vi "GUI_General_Camera.vi"() -> ()   [LabVIEW 2013]
uses:
  <vilib>/vision/NI_Vision_Development_Module.lvlib
  Shared/MySQL/Preset Query Enum.ctl
  <vilib>/Utility/miscctls.llb/LVRectTypeDef.ctl
panel:
  in  "resize":bool
  in  "Tab Control":T1(tab)
  in  "Maximize!!":bool
  out "Max Counts":dbl(slide) scale=0.0..256.0
  in  "triggerdelay":dbl
  in  "trigger":bool
  in  "save":bool
  in  "exposure":dbl=0.52 caption="Exposure"
  in  "gain":dbl
  in  "shotnumber":i32=354
  in  "autoscale":bool
  in  "LogArray":bool
  in  "beep if sat.":bool
  in  "sat level":sgl=255.0
  in  "lowpass":bool
  in  "Size & Tolerance":T2={"X Size"=5, "Y Size"=5, "% Tolerance"=10}
  in  "hide controls":bool
  in  "ROI.OffsetY":dbl
  in  "ROI.OffsetX":dbl
  in  "ROI.Height":dbl
  in  "ROI.Width":dbl
  in  "MaxGUIPixel":dbl
  out "Centroid":cluster{"X Centroid":sgl, "Y Centroid":sgl} {"Y Centroid" format="%.2f"; "X Centroid" format="%.2f"}
  out "Y Resolution":i32
  out "X Resolution":i32
  out "Mean Value":sgl format="%.2f"
  out "GUIBinning":dbl
  in  "Target.Y":dbl
  in  "Target.X":dbl
  in  "draw Xhair":bool
  in  "size 2":cluster{"xhair size":dbl, "xhair size 2":dbl}={"xhair size"=20.0, "xhair size 2"=20.0} {"xhair size 2" min=0.0 max=0.0; "xhair size" min=0.0 max=0.0}
  out "Mean Value 2":sgl(graph)
  out "histogram":T3(graph)
  out "lineout":cluster{"x0":sgl, "dx":sgl, "Pixels Line":sgl[]}(graph)
  out "MaxCounts":dbl
  in  "FWHMx":dbl
  in  "FWHMy":dbl
  out "MeanCounts":dbl
  out "FWHMx (um)":dbl
  out "FWHMy (um)":dbl
  in  "SpatialCalibration":dbl
  in  "Analysis":bool
  out "analysis error":errorcluster
  out "top":i16
  out "left":i16
  out "Zoom changed":bool
  out "Zoom old":cluster{"X":sgl, "Y":sgl}
  out "ratio(h)":bool=TRUE
  out "fixsize":bool
  out "Change Ratio":cluster{"X":sgl, "Y":sgl}={"X"=1.6671598, "Y"=0.6151203}
  out "old Panel Bounds":T4={"Left"=105, "Top"=80, "Right"=781, "Bottom"=662}
  out "error (h)":bool
  in  "Main Tap":enum32{"IMAQ", "Network", "Internal", "Array"}(tab)
  out "Image (IMAQ)":T5(plugin-control)
  out "local Port":u16=65401
  out "Remote Host":string="192.168.10.157"
  out "port or service name":u16=65400
  in  "timeout ms (slow resp)":i32=500
  in  "reset":bool
  out "All Devices (h)":string[](array[string])
  out "centroidy":dbl
  out "fast ID (h)":refnum<k16>
  out "slow ID (h)":refnum<k16>
  out "error out":errorcluster
  out "connections (hidden)":variant[](array[variant])=[variant(refnum<k16> refnum), variant(refnum<k16> refnum)]
  in  "time to wait (main loop)":i32=200
  in  "time to wait (TCP)":i32=10
  out "Data String":string="exposure,0.520000\r\ntrigger,off\r\nsave,off\r\ngain,0.000000\r\n"
  in  "send":bool
  in  "localsavingpath":path
  out "centroidy":dbl
  out "Image (array)":dbl[][](graph)
  out "Device Name (h)":string="FakeCam1"
  out "stop":bool
  out "error message":string
  out "image connection":bool
  out "data connection ok":bool
  # "Trigger"
  # "Save"
  # "Data"
  # "Image"
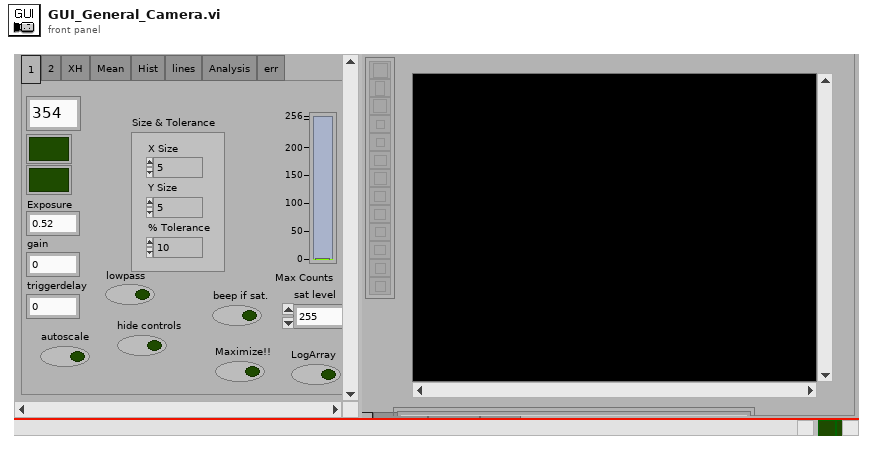
[diagram p1: front panel]
types:
  T1 = enum32{"1", "2", "XH", "Mean", "Hist", "lines", "Analysis", "err"}
  T2 = cluster{"X Size":i32, "Y Size":i32, "% Tolerance":i32}
  T3 = cluster{"Starting Value":sgl, "Incremental Value":sgl, "Histogram":u32[]}
  T4 = typedef "LVRectTypeDef.ctl" = cluster{"Left":i16, "Top":i16, "Right":i16, "Bottom":i16}
  T5 = typedef "IMAQ Image.ctl" = refnum<image>
  T6 = enum16{"Grayscale", "Binary", "Gradient", "Rainbow", "Temperature", "User Defined"}
  T7 = typedef "Preset Query Enum.ctl" = enum16{"Get Locations", "Get all IPs and MACs", "Get classes", "Get expt variables to set at scanstart for particular device", "Get expt devices and variables with start values", "Get expt devices and variables (with data to get)", "Get expt devices with data to get", "Get Expt devices and GUIs", "Get all devices basic properties", "Get Virtual Devices Core Info", "Get Expt names", "Get experiment basic properties", "Get experiment alarm variables", "Get MC Ports", "Get device network comm port", "Get devicetype lvclass path", "Get basic device properties", "Get Init Order", "Get all setable variables of a device", "Get device variable aliases", "Get force values of all settable variables", "Get all variables of a devicetype", "Get all variables of a device", "Get plotter details", "Get Saved Scans", "Get Scan Info", "GetGeneralGUIs", "Get expt for plotter", "Get plotter IDs from expt", "Get all devices", "Get all Virtual Devices", "Get all aliases", "Get variable and device info for Virtual Device", "GetItemLocatorIP", "Get IPs for GUIs", "Get DeviceType from Device", "GetLocalPortRange", "GetDevicePresetVariables", "Get Device Configuration", "GetAllPresetNames", "GetAllConfigurationNames", "GetPresetDeviceNames"}
  T8 = cluster{"Left":i32, "Top":i32, "Right":i32, "Bottom":i32}
  T9 = enum32{"Invalid", "Standard", "Closed", "Hidden", "Minimized", "Maximized"}
  T10 = typedef "Image Type" = u32
  T11 = cluster{"Global Rectangle":i32[], "Contours":cluster{"Contour Type":u32, "ROI Type":u32, "Points":i32[]}[]}
  T12 = typedef "EventTypDef.ctl" = refnum<user-event>
  T13 = typedef "LVBoundsTypeDef.ctl" = cluster{"Width":u32, "Height":u32}
  T14 = typedef "ROI Descriptor" = cluster{"Global Rectangle":i32[], "Contours":cluster{"ID":enum32{"External", "Internal"}, "Type":u32, "Coordinates":i32[]}[]}
  T15 = typedef "IMAQ Line" = cluster{"Start X":i32, "Start Y":i32, "End X":i32, "End Y":i32}
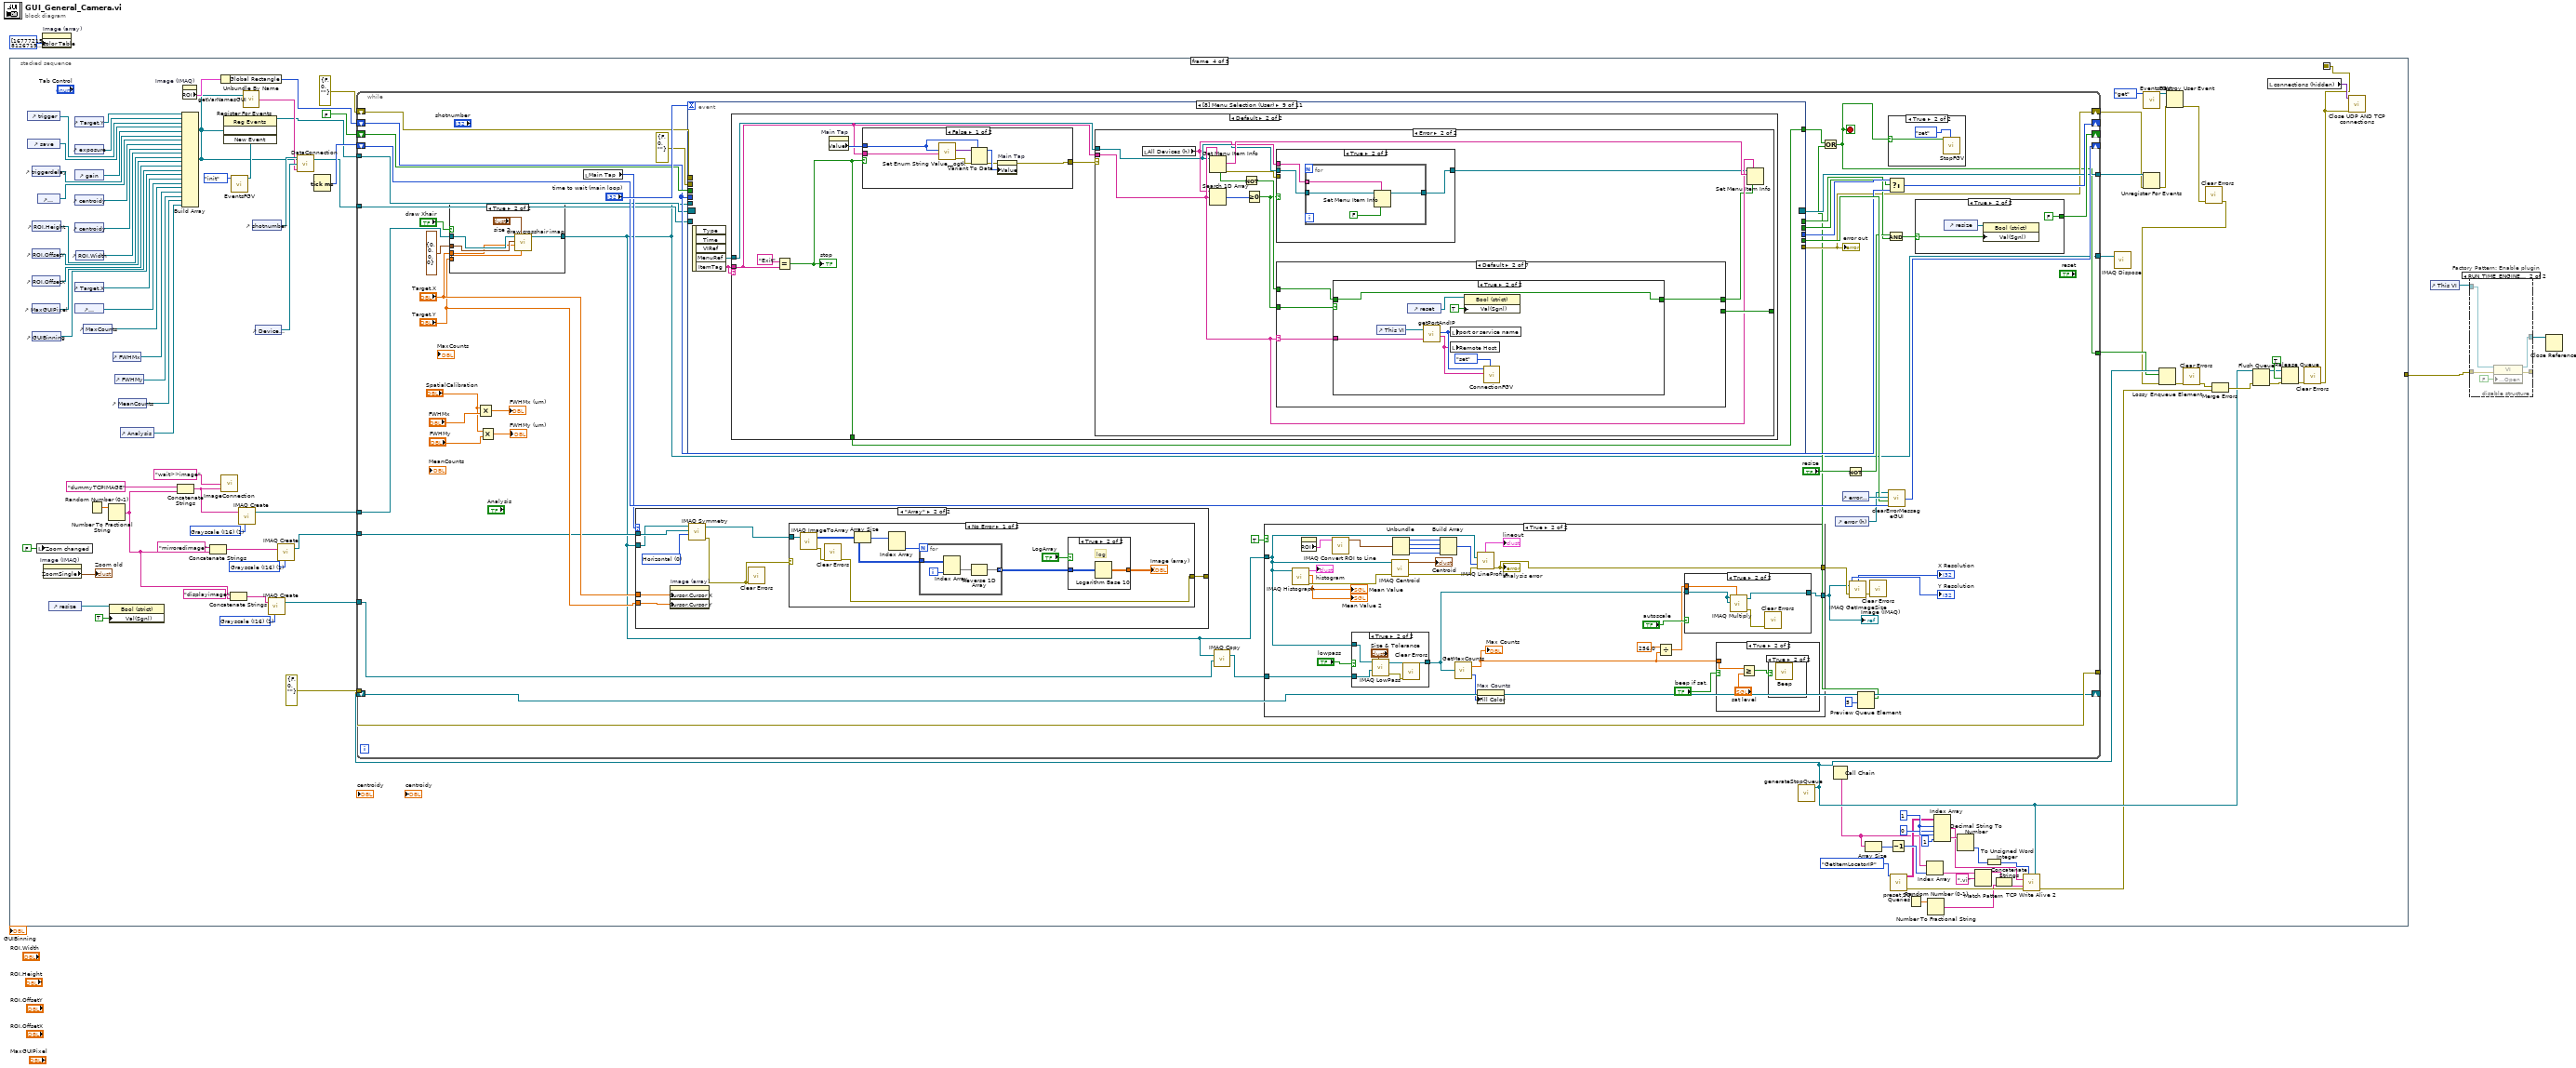
[diagram p0: block diagram]
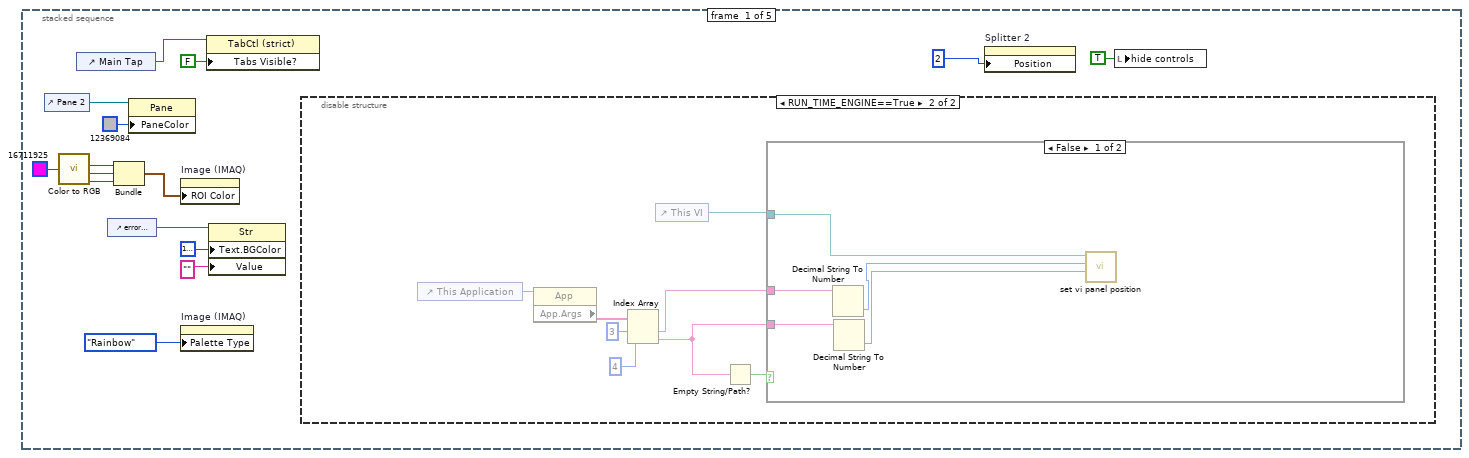
[diagram p3: hidden frame]
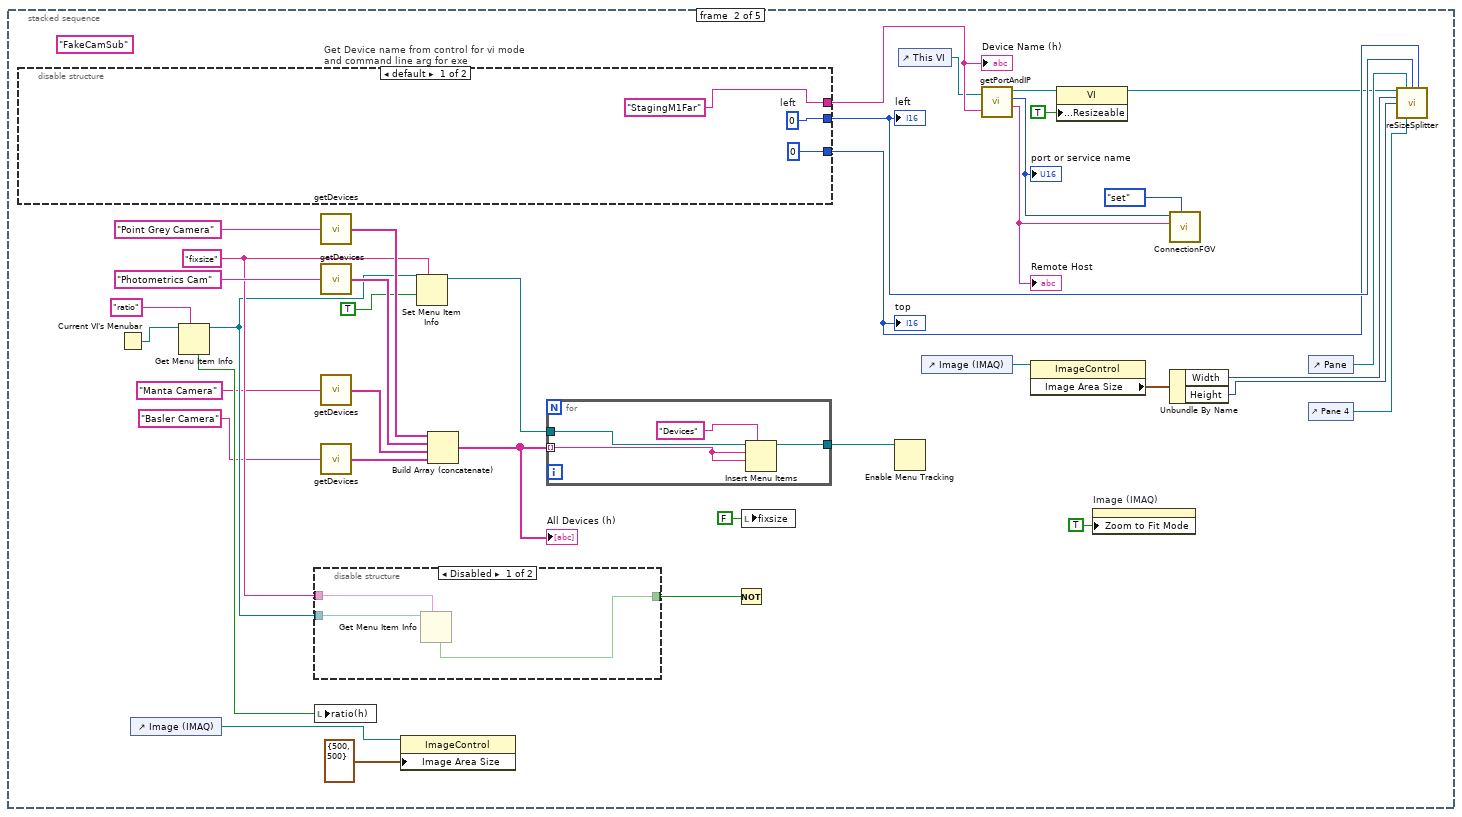
[diagram p6: hidden frame]
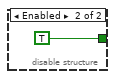
[diagram p7: hidden frame]
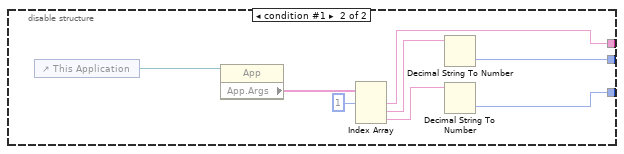
[diagram p8: hidden frame]
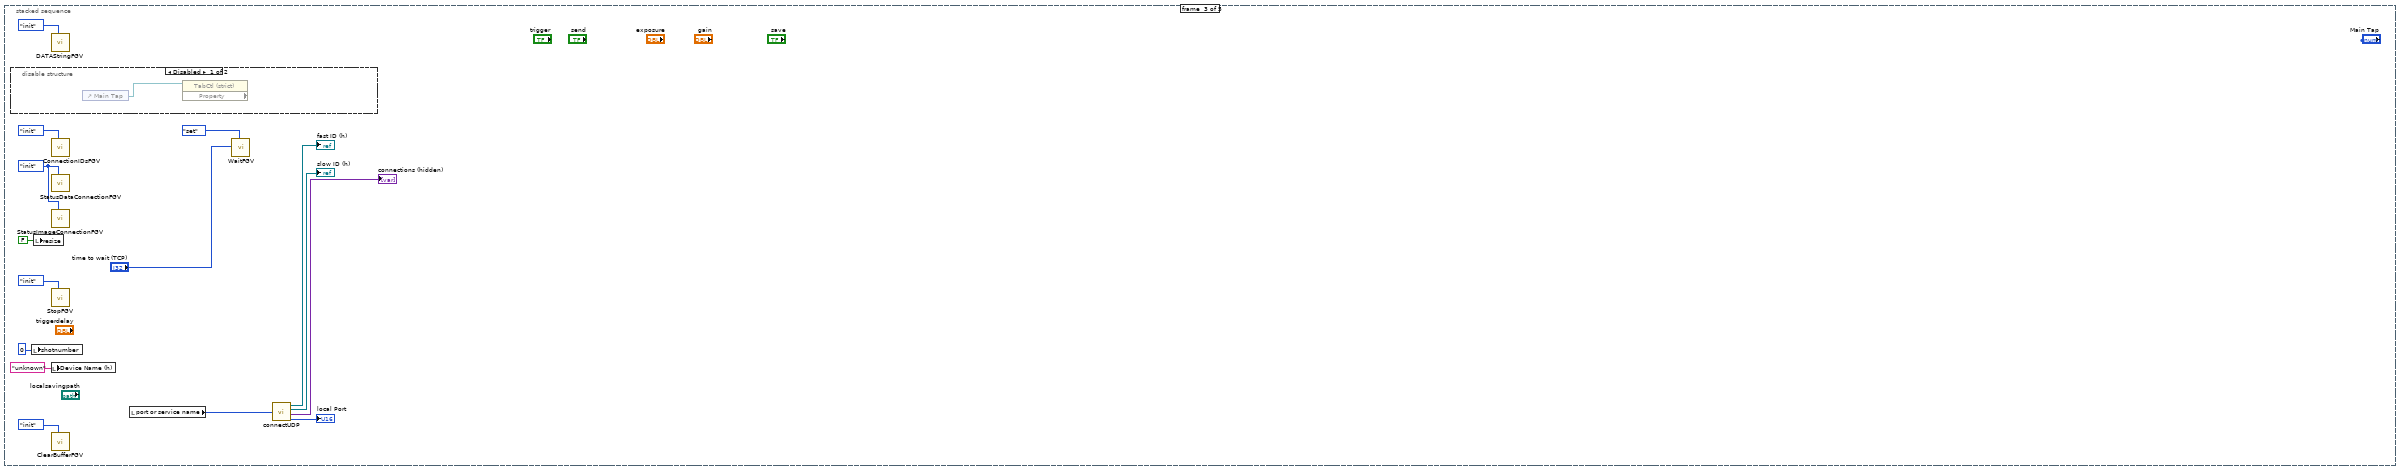
[diagram p9: hidden frame]
diagram:
  n1 = stacked-sequence {
    seq-local: [_ _ _ w140 _] -> [_ _ _ _ w550]
    tunnel: [_ _ _ _ w550] -> w2
    frame #0 {
      n2 = control-ref of="Pane 2"() -> (w14:refnum<vi>)
      n3 = call <vilib>:"Color to RGB.vi"("Color"=u32 16711925) -> ("R"=w10:u8, "G"=w9:u8, "B"=w8:u8)  [unwired: 1 out]
      n4 = control-ref of="Main Tap"() -> (w19:refnum<vi>)
      n5 = control-ref of="error message"() -> (w16:refnum<vi>)
      n6 = Bundle("R"=w10, "G"=w9, "B"=w8) -> (w7:cluster{"R":u8, "G":u8, "B":u8})  [unwired: 1 in]
      n7 = property class="Pane"(reference=w14, "PaneColor"=u32 12369084) -> ()  [unwired: 1 in, 2 out]
      n8 = property on="Image (IMAQ)" class="ImageControl"("ROI Color"=w7) -> ()  [unwired: 2 in, 2 out]
      n9 = property on="Image (IMAQ)" class="ImageControl"("Palette Type"=T6."Rainbow" ("Palette:Palette Type")) -> ()  [unwired: 2 in, 2 out]
      n10 = property class="TabCtl (strict)"(reference=w19, "Tabs Visible?"=FALSE) -> ()  [unwired: 1 in, 2 out]
      n11 = property class="Str"(reference=w16, "Text.BGColor"=u32 16777238, "Value"="") -> ()  [unwired: 1 in, 2 out]
      n12 = disable-structure shown="RUN_TIME_ENGINE==True" {
        frame condition #0 (active) {
        }
        frame condition #1 {
          n13 = control-ref of="This Application"() -> (w20:refnum<vi>)
          n14 = property class="App"(reference=w20) -> ("App.Args"=w27:string[])  [unwired: 1 in, 2 out]
          n15 = Index Array(array=w27, index #1=3 ("index"), index #2=4 ("index")) -> (element #1=w24:string, element #2=w23:string)
          n16 = control-ref of="This VI"() -> (w21:refnum<vi>)
          n17 = Empty String/Path?(string/path=w23) -> (empty?=w22:bool)
          n18 = case shown="False" w22 {
            tunnel: w24 -> [w32 _]
            tunnel: w21 -> [w28 _]
            tunnel: w23 -> [w29 _]
            frame False {
              n19 = Decimal String To Number(string=w32) -> (number=w31:i32)  [unwired: 2 in, 1 out]
              n20 = Decimal String To Number(string=w29) -> (number=w30:i32)  [unwired: 2 in, 1 out]
              n21 = call "set vi panel position.vi"("top"=w30, "left"=w31, "This VI"=w28) -> ()  [unwired: 7 in, 2 out]
            }
            frame True {
            }
          }
        }
      }
      n22 = property on="Splitter 2" class="Splitter"("Position"=2 ("Position:Left")) -> ()  [unwired: 2 in, 2 out]
      n23 = local write "hide controls"(TRUE ("hide controls")) -> ()
    }
    frame #1 {
      (unwired) "FakeCamSub" ("Device Class")
      w42 = "fixsize" ("item tag")
      n24 = disable-structure "Get Device name from control for vi mode\nand command line arg for exe" shown="default" {
        disable-tunnel: ["StagingM1Far" ("Device Name for vi mode") w86] -> w57
        disable-tunnel: [w80 w83] -> w62
        disable-tunnel: [i16 0 ("left") w82] -> w61
        frame condition #0 (active) {
          w80 = i16 0  # left
        }
        frame condition #1 {
          n25 = control-ref of="This Application"() -> (w89:refnum<vi>)
          n26 = property class="App"(reference=w89) -> ("App.Args"=w88:string[])  [unwired: 1 in, 2 out]
          n27 = Index Array(array=w88, index #1=1 ("index")) -> (element #1=w86:string, element #2=w85:string, element #3=w84:string)  [unwired: 2 in]
          n28 = Decimal String To Number(string=w85) -> (number=w83:i32)  [unwired: 2 in, 1 out]
          n29 = Decimal String To Number(string=w84) -> (number=w82:i32)  [unwired: 2 in, 1 out]
        }
      }
      "Device Name (h)" <- w57
      "left" <- w62
      "top" <- w61
      n30 = Current VI's Menubar() -> (w64:refnum<k9>)
      n31 = control-ref of="Image (IMAQ)"() -> (w45:refnum<vi>)
      n32 = Get Menu Item Info(7:"ratio" ("item tag"), 11:w64) -> (3:w41:refnum<k9>, 4:w63:bool)  [unwired: 1 in, 5 out]
      n33 = disable-structure shown="Disabled" {
        disable-tunnel: [w73 TRUE] -> w60
        disable-tunnel: w42 -> [w72 _]
        disable-tunnel: w41 -> [w71 _]
        frame Disabled {
          n34 = Get Menu Item Info(7:w72, 11:w71) -> (4:w73:bool)  [unwired: 1 in, 6 out]
        }
        frame Enabled {
        }
      }
      n35 = local write "ratio(h)"(w63) -> ()
      n36 = call "getDevices.vi"("Device Class"="Point Grey Camera") -> ("All Devices"=w48:string[])
      n37 = call "getDevices.vi"("Device Class"="Photometrics Cam") -> ("All Devices"=w47:string[])
      n38 = call "getDevices.vi"("Device Class"="Manta Camera") -> ("All Devices"=w37:string[])
      n39 = call "getDevices.vi"("Device Class"="Basler Camera") -> ("All Devices"=w35:string[])
      n40 = property class="ImageControl"(reference=w45, "Image Area Size"=cluster{"Width":u32, "Height":u32} {"Width"=500, "Height"=500} ("Image Area:Size:All Elements")) -> ()  [unwired: 1 in, 2 out]
      n41 = Set Menu Item Info(7:w42, 9:TRUE ("enabled"), 11:w41) -> (3:w40:refnum<k9>)  [unwired: 4 in, 1 out]
      n42 = Build Array (concatenate)(w48, w47, w37, w35) -> (w46:string[])
      "All Devices (h)" <- w46
      n43 = for {
        tunnel: w40 -> [w78]
        tunnel: [w77] -> w58
        tunnel: w46 -> [w75] mode=indexing
        n44 = Insert Menu Items(5:"Devices" ("menu tag"), 7:w75, 8:w75, 9:w78) -> (3:w77:refnum<k9>)  [unwired: 2 in, 2 out]
      }
      n45 = Not(x=w60) -> ()  [unwired: 1 out]
      n46 = local write "fixsize"(FALSE ("fixsize")) -> ()
      n47 = Enable Menu Tracking(4:w58) -> ()  [unwired: 2 in, 2 out]
      n48 = control-ref of="This VI"() -> (w56:refnum<vi>)
      n49 = control-ref of="Image (IMAQ)"() -> (w70:refnum<vi>)
      n50 = call "getPortAndIP.vi"("This Vi"=w56, "Device Name"=w57) -> ("reference out"=w55:refnum<vi>, "port or service name"=w52:u16, "Remote Host"=w51:string)  [unwired: 1 in]
      "port or service name" <- w52
      "Remote Host" <- w51
      n51 = property class="ImageControl"(reference=w70) -> ("Image Area Size"=w69:cluster{"Width":u32, "Height":u32})  [unwired: 1 in, 2 out]
      n52 = property class="VI"(reference=w55, "Front Panel.Resizeable"=TRUE ("Front Panel Window:Resizable")) -> (reference out=w54:refnum<vi>)  [unwired: 1 in, 1 out]
      n53 = property on="Image (IMAQ)" class="ImageControl"("Zoom to Fit Mode"=TRUE) -> ()  [unwired: 2 in, 2 out]
      n54 = call "ConnectionFGV.vi"("command"=enum16{"get", "set", "init"}."set", "Remote Host in"=w51, "port or service name in"=w52) -> ()  [unwired: 7 in, 2 out]
      n55 = Unbundle By Name(w69) -> ("Width"=w68:u32, "Height"=w67:u32)
      n56 = control-ref of="Pane"() -> (w66:refnum<vi>)
      n57 = control-ref of="Pane 4"() -> (w59:refnum<vi>)
      n58 = call "reSizeSplitter.vi"("this vi"=w54, "pane"=w66, "left"=w62, "top"=w61, "Width"=w68, "Height"=w67, "pane2"=w59) -> ()  [unwired: 8 in, 1 out]
    }
    frame #2 {
      w100 = enum16{"get", "set", "init"}."init" ("Command")
      n59 = disable-structure shown="Disabled" {
        frame Disabled {
          n60 = control-ref of="Main Tap"() -> (w105:refnum<vi>)
          n61 = property class="TabCtl (strict)" props=[](reference=w105) -> ()  [unwired: 1 in, 3 out]
        }
        frame Enabled {
        }
      }
      n62 = local write "shotnumber"(0 ("shotnumber")) -> ()
      n63 = local write "resize"(FALSE ("resize")) -> ()
      n64 = call "DATAStringFGV.vi"("Command"=enum16{"get", "set", "init"}."init") -> ()  [unwired: 9 in, 2 out]
      n65 = call "ConnectionIDsFGV.vi"("Command"=enum16{"add", "get", "init"}."init") -> ()  [unwired: 10 in, 1 out]
      n66 = call "StatusDataConnectionFGV.vi"("Command"=w100) -> ()  [unwired: 10 in, 1 out]
      n67 = call "StatusImageConnectionFGV.vi"("Command"=w100) -> ()  [unwired: 10 in, 1 out]
      n68 = call "StopFGV.vi"("Command"=enum16{"set", "get", "init"}."init") -> ()  [unwired: 9 in, 2 out]
      n69 = local write "Device Name (h)"("unknown" ("Device Name")) -> ()
      n70 = call "ClearBufferFGV.vi"("Command"=enum16{"set", "get", "init"}."init") -> ()  [unwired: 10 in, 1 out]
      n71 = local read "port or service name"() -> (w102:u16)
      n72 = call "WaitFGV.vi"("Command"=enum16{"get", "set", "init"}."set", "milliseconds to wait"="time to wait (TCP)") -> ()  [unwired: 9 in, 1 out]
      n73 = call "connectUDP.vi"("port or service name NOT USED"=w102) -> ("fast ID (h)"=→"fast ID (h)":refnum<k16>, "slow ID (h)"=→"slow ID (h)":refnum<k16>, "connections (hidden)"=→"connections (hidden)":variant[], "local Port"=→"local Port":u16)
    }
    frame #3 {
      w110 = T10 1 items=["Grayscale (U8)", "Grayscale (I16)", "Grayscale (SGL)", "Complex (CSG)", "RGB (U32)", "HSL (U32)", "RGB (U64)", "Grayscale (U16)"] ("Image Type")
      w114 = T10 1 items=["Grayscale (U8)", "Grayscale (I16)", "Grayscale (SGL)", "Complex (CSG)", "RGB (U32)", "HSL (U32)", "RGB (U64)", "Grayscale (U16)"] ("Image Type")
      w129 = 1 ("index (row)")
      w196 = T10 1 items=["Grayscale (U8)", "Grayscale (I16)", "Grayscale (SGL)", "Complex (CSG)", "RGB (U32)", "HSL (U32)", "RGB (U64)", "Grayscale (U16)"] ("Image Type")
      n74 = control-ref of="trigger"() -> (w189:refnum<vi>)
      n75 = control-ref of="save"() -> (w187:refnum<vi>)
      n76 = control-ref of="triggerdelay"() -> (w185:refnum<vi>)
      n77 = control-ref of="ROI.OffsetY"() -> (w159:refnum<vi>)
      n78 = control-ref of="ROI.OffsetX"() -> (w158:refnum<vi>)
      n79 = control-ref of="MaxGUIPixel"() -> (w157:refnum<vi>)
      n80 = control-ref of="ROI.Height"() -> (w160:refnum<vi>)
      n81 = control-ref of="GUIBinning"() -> (w156:refnum<vi>)
      n82 = local write "Zoom changed"(FALSE ("Zoom changed")) -> ()
      n83 = control-ref of="localsavingpath"() -> (w181:refnum<vi>)
      n84 = property on="Image (IMAQ)" class="ImageControl"() -> ("ZoomSingle"=→"Zoom old":cluster{"X":sgl, "Y":sgl})  [unwired: 2 in, 2 out]
      n85 = control-ref of="resize"() -> (w171:refnum<vi>)
      n86 = control-ref of="Target.Y"() -> (w154:refnum<vi>)
      n87 = control-ref of="exposure"() -> (w188:refnum<vi>)
      n88 = control-ref of="gain"() -> (w186:refnum<vi>)
      n89 = control-ref of="centroidy"() -> (w180:refnum<vi>)
      n90 = control-ref of="centroidy"() -> (w174:refnum<vi>)
      n91 = control-ref of="Target.X"() -> (w155:refnum<vi>)
      n92 = control-ref of="SpatialCalibration"() -> (w153:refnum<vi>)
      n93 = control-ref of="ROI.Width"() -> (w161:refnum<vi>)
      n94 = control-ref of="MaxCounts"() -> (w152:refnum<vi>)
      n95 = Random Number (0-1)() -> (number: 0 to 1=w194:dbl)
      n96 = Number To Fractional String(number=w194) -> (F-format string=w106:string)  [unwired: 3 in]
      n97 = property class="Bool (strict)"(reference=w171, "Val(Sgnl)"=TRUE ("Value (Signaling)")) -> ()  [unwired: 1 in, 2 out]
      n98 = control-ref of="FWHMx"() -> (w151:refnum<vi>)
      n99 = control-ref of="FWHMy"() -> (w150:refnum<vi>)
      n100 = control-ref of="MeanCounts"() -> (w149:refnum<vi>)
      n101 = control-ref of="Analysis"() -> (w148:refnum<vi>)
      n102 = Concatenate Strings("dummyTCPIMAGE" ("Image Name"), w106) -> (w192:string)
      n103 = Build Array(w154, w188, w189, w187, w186, w185, w181, w180, w174, w161, w160, w159, w158, w157, w156, w155, w153, w152, w151, w150, w149, w148) -> (w168:refnum<vi>[])
      n104 = property on="Image (IMAQ)" class="ImageControl"() -> ("ROI"=w179:T11)  [unwired: 2 in, 2 out]
      n105 = Concatenate Strings("mirroredimage" ("string"), w106) -> (w112:string)
      n106 = Unbundle By Name(w179) -> ("Global Rectangle"=w178:i32[])
      n107 = call "ImageConnection.vi"("Image Name"=w192, "Image Subscriber list"="wait>>image") -> ()  [unwired: 2 in]
      n108 = Concatenate Strings("displayimage" ("string"), w106) -> (w108:string)
      n109 = call "EventsFGV.vi"("Command"=enum16{"get", "init"}."init") -> ("New Event"=w169:T12)  [unwired: 9 in, 1 out]
      n110 = register-events(w168, w169) -> (reference out=w167:refnum<event-registration>)  [unwired: 2 in, 1 out]
      n111 = call "IMAQ Create"("Image Name"=w192, "Image Type"=w196) -> ("New Image"=w195:T5)  [unwired: 3 in, 1 out]
      n112 = call "getVarNamesGUI.vi"("Array"=w168) -> ("String"=w173:string)  [unwired: 1 in]
      n113 = control-ref of="shotnumber"() -> (w176:refnum<vi>)
      n114 = control-ref of="Device Name (h)"() -> (w175:refnum<vi>)
      n115 = call "IMAQ Create"("Image Name"=w108, "Image Type"=w110) -> ("New Image"=w107:T5)  [unwired: 3 in, 1 out]
      n116 = call "IMAQ Create"("Image Name"=w112, "Image Type"=w114) -> ("New Image"=w111:T5)  [unwired: 3 in, 1 out]
      n117 = call "DataConnection.vi"("Subscriber list"=w173, "Device Name (h)"=w175, "shotnumber"=w176) -> ()
      n118 = Tick Count (ms)() -> (millisecond timer value=w182:u32)
      n119 = call "generateStopQueue.vi"() -> ("STOP Queue out"=w123:refnum<queue>)  [unwired: 10 in, 1 out]
      n120 = while {
        shift-right: [w226] -> w164
        shift-left: errorcluster {"status"=FALSE, "code"=0, "source"=""} ("error out") -> [w246]
        tunnel: w195 -> [w225]
        tunnel: [w201] -> w197
        tunnel: w168 -> [w233]
        shift-right: [w232] -> _
        shift-left: FALSE -> [w245]
        shift-right: [w244] -> _
        shift-left: w182 -> [w243]
        shift-right: [w238] -> _
        shift-left: w178 -> [w237]
        tunnel: w167 -> [w234]
        tunnel: [w227] -> w166
        tunnel: errorcluster {"status"=FALSE, "code"=0, "source"=""} ("error out") -> [w213]
        tunnel: [w213] -> _
        tunnel: [w209] -> w120
        shift-right: [w212] -> _
        shift-left: w123 -> [w214]
        tunnel: w111 -> [w207]
        tunnel: w107 -> [w200]
        stop <- w209 stop-if-true
        n121 = case shown="True" "draw Xhair" {
          tunnel: "Target.Y" -> [_ w291]
          tunnel: "Target.X" -> [_ w292]
          tunnel: w225 -> [w289 w295]
          tunnel: [w289 w293] -> w201
          tunnel: T8 {"Left"=0, "Top"=0, "Right"=0, "Bottom"=0} ("Bounding Rectangle") -> [_ w294]
          frame False {
          }
          frame True {
            n122 = call "draw crosshair imaq.vi"(6:w291, "clear overlay"="size 2", "Crosshair"=w292, "Bounding Rectangle"=w294, "image in"=w295) -> ("image out"=w293:T5)  [unwired: 5 in, 1 out]
          }
        }
        n123 = Multiply(x="SpatialCalibration", y="FWHMx") -> (x*y=→"FWHMx (um)":dbl)
        n124 = Multiply(x="SpatialCalibration", y="FWHMy") -> (x*y=→"FWHMy (um)":dbl)
        n125 = local read "Main Tap"() -> (w240:enum32{"IMAQ", "Network", "Internal", "Array"})
        n126 = case shown="\"Array\"" w240 {
          tunnel: w201 -> [_ w306]
          tunnel: "Target.X" -> [_ w309]
          tunnel: "Target.Y" -> [_ w308]
          tunnel: w207 -> [_ w307]
          tunnel: [_ w302] -> _
          frame "IMAQ", Default {
          }
          frame "Array" {
            w305 = u32 0 items=["Horizontal", "Vertical", "Central", "1st Diagonal", "2nd Diagonal"] ("Type of Symmetry")
            n127 = property on="Image (array)" class="IntGraph (strict)"("Cursor.Cursor X"=w309, "Cursor.Cursor Y"=w308) -> ()  [unwired: 2 in, 2 out]
            n128 = call "IMAQ Symmetry"("Type of Symmetry"=w305, "Image Dst"=w307, "Image Src"=w306) -> ("error out"=w303:errorcluster, "Image Dst Out"=w304:T5)  [unwired: 2 in]
            n129 = call <vilib>:"Clear Errors.vi"("error in (no error)"=w303) -> ()  [unwired: 6 in, 1 out]
            n130 = case shown="No Error" w303 {
              tunnel: w304 -> [w311 _]
              tunnel: [w310 _] -> w302
              frame No Error {
                n131 = call "IMAQ ImageToArray"("Image"=w311) -> ("error out"=w318:errorcluster, "Image Pixels (I16)"=w312:i16[][])  [unwired: 3 in, 3 out]
                n132 = call <vilib>:"Clear Errors.vi"("error in (no error)"=w318) -> ("error out"=w310:errorcluster)  [unwired: 6 in]
                n133 = Array Size(array=w312) -> (size(s)=w317:i32[])
                n134 = Index Array(array=w317) -> (element #2=w316:i32)  [unwired: 2 in, 1 out]
                n135 = for {
                  N: w316 -> [_]
                  tunnel: w312 -> [w325]
                  tunnel: [w323] -> w314 mode=indexing
                  i -> [w322]
                  n136 = Index Array(array=w325, index (col)=w322) -> (element=w324:i16[])  [unwired: 1 in]
                  n137 = Reverse 1D Array(array=w324) -> (reversed array=w323:i16[])
                }
                n138 = case shown="True" "LogArray" {
                  tunnel: w314 -> [w319 w321]
                  tunnel: [w319 w320] -> w313
                  frame False {
                  }
                  frame True {
                    # "log"
                    n139 = Logarithm Base 10(1:w321) -> (0:w320:dbl[][])
                  }
                }
                "Image (array)" <- w313
              }
              frame Error {
              }
            }
          }
        }
        n140 = event shown="[8] Menu Selection (User)" {
          selector: w234 -> [_ _ _ _ _ _ _ _ _ _ _]
          dyn-events: [_ _ _ _ _ _ _ _ _ _ _] -> w227
          timeout: "time to wait (main loop)" -> [_ _ _ _ _ _ _ _ _ _ _]
          tunnel: [w331 _ _ _ _ _ _ w449 _ _ _] -> w226
          tunnel: errorcluster {"status"=FALSE, "code"=0, "source"=""} ("error out") -> [w333 _ _ _ _ _ _ _ _ _ _]
          tunnel: w246 -> [_ _ _ _ _ _ _ w449 _ _ _]
          tunnel: [TRUE _ _ _ _ _ _ _ _ _ _] -> w241
          tunnel: [_ _ _ _ _ _ _ _ w452 _ _] -> w211
          tunnel: w245 -> [_ _ _ _ _ _ _ _ _ _ _]
          tunnel: [_ w341 w353 TRUE _ _ _ _ _ _ _] -> w229
          tunnel: [_ _ _ _ _ _ _ _ _ _ w526] -> w239
          tunnel: w237 -> [_ _ _ _ _ _ _ _ _ _ w527]
          tunnel: [_ _ _ _ _ _ _ _ _ _ w525] -> w236
          tunnel: w201 -> [_ _ _ _ _ _ w393 _ _ _ w528]
          tunnel: w233 -> [_ _ _ _ _ w383 _ _ _ _ _]
          event Value Change {
            n141 = event-data() -> ("CtlRef"=w328:refnum<vi>, "NewVal"=w327:variant)  [unwired: 1 in, 3 out]
            n142 = call "SendCommandEvent.vi"("timeout ms (slow resp)"="timeout ms (slow resp)", "error out 2"=w333, "NewVal"=w327, "CtlRef"=w328) -> ("error out"=w331:errorcluster, "error (h)"=→"error (h)":bool, "error message"=→"error message":string)  [unwired: 4 in, 1 out]
          }
          event Panel Resize {
            n143 = event-data() -> ("Time"=w339:u32, "OldBnds"=w336:T4, "NewBnds"=w335:T4)  [unwired: 1 in, 4 out]
            n144 = Tick Count (ms)() -> (millisecond timer value=w340:u32)
            n145 = Subtract(x=w340, y=w339) -> (x-y=w338:u32)
            n146 = Equal?(x=w336, y=w335) -> (x = y?=w334:bool)
            n147 = Greater?(x=w338, y=u32 1000) -> ()  [unwired: 1 out]
            n148 = case shown="True" w334 {
              tunnel: w335 -> [w347 _]
              tunnel: [TRUE _] -> w341
              tunnel: w336 -> [_ _]
              frame True {
                n149 = local read "old Panel Bounds"() -> (w342:T4)
                n150 = call "getWidthAndHight.vi"("OldBnds"=w342) -> ("output cluster"=w345:cluster{"X":sgl, "Y":sgl})
                n151 = call "getWidthAndHight.vi"("OldBnds"=w347) -> ("output cluster"=w344:cluster{"X":sgl, "Y":sgl})
                n152 = Divide(x=w345, y=w344) -> (x/y=→"Change Ratio":cluster{"X":sgl, "Y":sgl})
              }
              frame False {
              }
            }
          }
          event "Maximize!!": Value Change {
            n153 = event-data() -> ()  [unwired: 1 in, 5 out]
            n154 = property class="VI"() -> (error out=w348:errorcluster, "Front Panel.PanelBounds"=w349:T4)  [unwired: 2 in, 1 out]
            n155 = case shown="True" "Maximize!!" {
              tunnel: w349 -> [w363 w367]
              tunnel: [w363 w367] -> w351
              tunnel: [_ w366] -> w350
              tunnel: w348 -> [_ w364]
              frame False {
              }
              frame True {
                n156 = local write "Maximize!!"(FALSE ("Maximize!!")) -> ()
                n157 = property class="VI"(error in=w364, "Front Panel Window:State"=T9."Maximized") -> (error out=w366:errorcluster)  [unwired: 1 in, 1 out]
                n158 = Wait (ms)(milliseconds to wait=u32 200) -> ()  [unwired: 1 out]
              }
            }
            n159 = case shown="True" TRUE {
              tunnel: [TRUE _] -> w353
              tunnel: w351 -> [w359 _]
              tunnel: w350 -> [w357 _]
              frame True {
                n160 = property class="VI"(error in=w357) -> ("Front Panel.PanelBounds"=w358:T4)  [unwired: 1 in, 2 out]
                n161 = call "getWidthAndHight.vi"("OldBnds"=w359) -> ("output cluster"=w362:cluster{"X":sgl, "Y":sgl})
                n162 = call "getWidthAndHight.vi"("OldBnds"=w358) -> ("output cluster"=w361:cluster{"X":sgl, "Y":sgl})
                n163 = Divide(x=w362, y=w361) -> (x/y=w355:cluster{"X":sgl, "Y":sgl})
                n164 = local write "Change Ratio"(w355) -> ()
                n165 = local write "resize"(TRUE ("resize")) -> ()
              }
              frame False {
              }
            }
          }
          event "hide controls": Value Change {
            n166 = event-data() -> ("NewVal"=w373:bool)  [unwired: 1 in, 4 out]
            n167 = case shown="True" w373 {
              tunnel: [367 ("Position:Left") 2 ("Position:Left")] -> w372
              frame False {
              }
              frame True {
              }
            }
            n168 = local write "Change Ratio"(cluster{"X":sgl, "Y":sgl} {"X"=1.0, "Y"=1.0} ("Change Ratio")) -> ()
            n169 = property on="Splitter 2" class="Splitter"("Position"=w372) -> ()  [unwired: 2 in, 2 out]
          }
          event "reset": Value Change {
            n170 = event-data() -> ()  [unwired: 1 in, 5 out]
            n171 = flat-sequence {
              frame #0 {
                n172 = local read "connections (hidden)"() -> (w377:variant[])
                n173 = call "Close UDP AND TCP connections.vi"("appended array"=w377) -> ()  [unwired: 7 in]
              }
              frame #1 {
                n174 = call "ConnectionFGV.vi"("command"=enum16{"get", "set", "init"}."get") -> ("port or service name out"=w379:u16)  [unwired: 9 in, 1 out]
                n175 = call "connectUDP.vi"("port or service name NOT USED"=w379) -> ("connections (hidden)"=w378:variant[])  [unwired: 3 out]
                n176 = local write "connections (hidden)"(w378) -> ()
              }
              frame #2 {
                n177 = Wait (ms)(milliseconds to wait=u32 500) -> ()  [unwired: 1 out]
              }
              frame #3 {
                n178 = property on="Image (IMAQ)" class="ImageControl"("Zoom to Fit Mode"=TRUE) -> ()  [unwired: 2 in, 2 out]
              }
            }
            n179 = local write "reset"(FALSE ("reset")) -> ()
          }
          event User Event {
            n180 = event-data() -> ("EventEnum"=w384:enum16{"new data", "connection status update"})  [unwired: 1 in, 3 out]
            n181 = case shown="\"new data\", Default" w384 {
              tunnel: w383 -> [w386 _]
              frame "new data", Default {
                n182 = call "DATAStringFGV.vi"("Command"=enum16{"get", "set", "init"}."get") -> ("Data String out"=w385:string)  [unwired: 9 in, 1 out]
                "Data String" <- w385
                n183 = call "Update Indicators (Data String to ref array).vi"("Array"=w386, "Data String"=w385) -> ()  [unwired: 12 in, 2 out]
              }
              frame "connection status update" {
                n184 = call "StatusDataConnectionFGV.vi"("Command"=enum16{"get", "set", "init"}."get") -> ("Data Connection out"=→"image connection":bool)  [unwired: 10 in]
                n185 = call "StatusImageConnectionFGV.vi"("Command"=enum16{"get", "set", "init"}."get") -> ("Image Connection out"=→"data connection ok":bool)  [unwired: 10 in]
              }
            }
          }
          event "resize": Value Change {
            n186 = event-data() -> ()  [unwired: 1 in, 5 out]
            n187 = call "GetImageRes.vi"("Image"=w393) -> ("valid Image"=w392:bool)  [unwired: 6 in, 4 out]
            n188 = case shown="True" w392 {
              tunnel: w393 -> [_ w402]
              frame False {
                n189 = local write "resize"(FALSE ("resize")) -> ()
              }
              frame True {
                w410 = 0.0 ("lower limit")
                n190 = local write "resize"(FALSE ("resize")) -> ()
                n191 = local read "Change Ratio"() -> (w426:cluster{"X":sgl, "Y":sgl})
                n192 = property on="Image (IMAQ)" class="ImageControl"() -> (error out=w397:errorcluster, "ZoomSingle"=w427:cluster{"X":sgl, "Y":sgl})  [unwired: 2 in, 1 out]
                n193 = Divide(x=w427, y=w426) -> (x/y=w396:cluster{"X":sgl, "Y":sgl})
                n194 = flat-sequence {
                  tunnel: [w431] -> w395
                  tunnel: w396 -> [w429]
                  tunnel: [w428] -> w398
                  tunnel: w397 -> [w428]
                  frame #0 {
                    n195 = control-ref of="Image (IMAQ)"() -> (w433:refnum<vi>)
                    n196 = local read "ratio(h)"() -> (w432:bool)
                    n197 = call "updateZoom.vi"("Zoom old"=w429, "ratio(h)"=w432, "update Zoom"=TRUE, "imageRef"=w433) -> ("Zoom out"=w431:cluster{"X":sgl, "Y":sgl})  [unwired: 7 in]
                  }
                }
                n198 = local write "Zoom old"(w395) -> ()
                n199 = call "GetImageRes.vi"("error in (no error)"=w398, "Image"=w402) -> ("Image Area:Size:All Elements"=w403:cluster{"Width":u32, "Height":u32}, "Y Resolution"=w404:i32, "X Resolution"=w405:i32)  [unwired: 5 in, 2 out]
                n200 = control-ref of="Image (IMAQ)"() -> (w417:refnum<vi>)
                n201 = Multiply(x=w403, y=w395) -> (x*y=w425:cluster{sgl, sgl})
                n202 = control-ref of="This VI"() -> (w406:refnum<vi>)
                n203 = local read "fixsize"() -> (w418:bool)
                n204 = case shown="False" w418 {
                  tunnel: w425 -> [w437 _]
                  tunnel: w406 -> [w434 w448]
                  tunnel: [w440 w448] -> w423
                  tunnel: w417 -> [w439 _]
                  frame False {
                    w435 = i16 0 ("left")
                    n205 = property class="ImageControl"(reference=w439, "Image Area Size"=w437) -> ()  [unwired: 1 in, 2 out]
                    n206 = disable-structure shown="Enabled" {
                      disable-tunnel: w437 -> [w446 w447]
                      disable-tunnel: [w445 w447] -> w436
                      frame Enabled {
                        n207 = Subtract(x=w446, y=cluster{sgl, sgl} {40.0, 70.0}) -> (x-y=w445:cluster{sgl, sgl})
                      }
                      frame Disabled {
                      }
                    }
                    n208 = Unbundle(w437) -> (w442:sgl, w443:sgl)
                    n209 = property on="Image (array)" class="IntGraph (strict)"("Plot Area Size"=w436) -> ()  [unwired: 2 in, 2 out]
                    n210 = control-ref of="Pane"() -> (w441:refnum<vi>)
                    n211 = control-ref of="Pane 4"() -> (w438:refnum<vi>)
                    n212 = call "reSizeSplitter.vi"("this vi"=w434, "pane"=w441, "left"=w435, "top"=w435, "Width"=w442, "Height"=w443, "pane2"=w438) -> ("reference out"=w440:refnum<vi>)  [unwired: 8 in]
                  }
                  frame True {
                  }
                }
                n213 = property class="VI"(reference=w423) -> (error out=w401:errorcluster, "Front Panel.PanelBounds"=w422:T4)  [unwired: 1 in, 1 out]
                "old Panel Bounds" <- w422
                n214 = property on="Image (array)" class="IntGraph (strict)"(error in=w401) -> (error out=w400:errorcluster, "Plot Area Size"=w416:T13, "XScale.Minimum"=w411:dbl, "YScale.Minimum"=w409:dbl)  [unwired: 1 in, 1 out]
                n215 = Unbundle By Name(w422) -> ("Right"=w421:i16, "Left"=w420:i16)
                n216 = Unbundle By Name(w416) -> ("Width"=w415:u32, "Height"=w413:u32)
                n217 = In Range and Coerce(upper limit=w404, x=w409, lower limit=w410) -> (coerced(x)=w408:dbl)  [unwired: 1 out]
                n218 = Subtract(x=w421, y=w420) -> (x-y=w419:i16)
                n219 = control-ref of="error message"() -> (w424:refnum<vi>)
                n220 = In Range and Coerce(upper limit=w405, x=w411, lower limit=w410) -> (coerced(x)=w412:dbl)  [unwired: 1 out]
                n221 = property class="Str"(reference=w424, "Width"=w419) -> ()  [unwired: 1 in, 2 out]
                n222 = Subtract(x=w415, y=w412) -> (x-y=w414:dbl)
                n223 = Subtract(x=w413, y=w409) -> (x-y=w407:dbl)
                n224 = property on="Image (array)" class="IntGraph (strict)"(error in=w400, "XScale.Minimum"=w412, "XScale.Maximum"=w414, "YScale.Minimum"=w408, "YScale.Maximum"=w407) -> ()  [unwired: 1 in, 2 out]
              }
            }
          }
          event Timeout {
            n225 = event-data() -> ()  [unwired: 1 in, 2 out]
          }
          event Menu Selection (User) {
            n226 = event-data() -> ("MenuRef"=w451:refnum<k9>, "ItemTag"=w450:string)  [unwired: 1 in, 3 out]
            n227 = case shown="Default" w450 {
              tunnel: [_ w458] -> w452
              tunnel: w450 -> [_ w456]
              tunnel: w451 -> [_ w455]
              frame "Controls" {
                n228 = local read "hide controls"() -> (w454:bool)
                n229 = Not(x=w454) -> (.not. x?=w453:bool)
                n230 = property on="hide controls" class="Bool (strict)"("Val(Sgnl)"=w453) -> ()  [unwired: 2 in, 2 out]
              }
              frame Default {
                n231 = Equal?(x="Exit", y=w456) -> (x = y?=w458:bool)
                "stop" <- w458
                n232 = property on="Main Tap" class="TabCtl (strict)"() -> ("Value"=w460:enum32{"IMAQ", "Network", "Internal", "Array"})  [unwired: 2 in, 2 out]
                n233 = case shown="False" w458 {
                  tunnel: w460 -> [w519 _]
                  tunnel: w456 -> [w518 _]
                  tunnel: [w515 errorcluster {"status"=FALSE, "code"=0, "source"=""} ("error out")] -> w457
                  frame False {
                    n234 = call <userlib>:"Set Enum String Value__ogtk.vi"("String Value"=w518, "Default Enum Value"=w519) -> ("error out"=w517:errorcluster, "Enum"=w521:variant)  [unwired: 8 in]
                    n235 = Variant To Data(error in=w517, type=w519, Variant=w521) -> (data=w520:enum32{"IMAQ", "Network", "Internal", "Array"}, error out=w516:errorcluster)
                    n236 = property on="Main Tap" class="TabCtl (strict)"(error in=w516, "Value"=w520) -> (error out=w515:errorcluster)  [unwired: 1 in, 1 out]
                  }
                  frame True {
                  }
                }
                n237 = case shown="Error" w457 {
                  tunnel: w455 -> [_ w464]
                  tunnel: w456 -> [_ w468]
                  tunnel: [_ w469] -> _
                  frame No Error {
                  }
                  frame Error {
                    n238 = local read "All Devices (h)"() -> (w466:string[])
                    n239 = Search 1D Array(1D array=w466, element=w468) -> (index of element=w467:i32)  [unwired: 1 in]
                    n240 = Get Menu Item Info(7:w468, 11:w464) -> (0:w465:errorcluster, 2:w471:string, 4:w472:bool)  [unwired: 1 in, 4 out]
                    n241 = Not(x=w472) -> (.not. x?=w470:bool)
                    n242 = Greater Or Equal To 0?(x=w467) -> (x >= 0?=w463:bool)
                    n243 = case shown="True" w463 {
                      tunnel: w466 -> [_ w476]
                      tunnel: w465 -> [_ _]
                      tunnel: w464 -> [w473 w475]
                      tunnel: [w473 w474] -> w462
                      frame False {
                      }
                      frame True {
                        n244 = for {
                          tunnel: w476 -> [w480] mode=indexing
                          tunnel: w475 -> [w478]
                          tunnel: [w477] -> w474
                          n245 = Set Menu Item Info(6:FALSE ("checked"), 7:w480, 11:w478) -> (3:w477:refnum<k9>)  [unwired: 4 in, 1 out]
                        }
                      }
                    }
                    n246 = case shown="Default" w468 {
                      selector: w468 -> [_ w486 _ _ w507 _ _]
                      tunnel: w470 -> [w481 w484 w497 _ _ _ w512]
                      tunnel: [_ _ TRUE _ _ _ _] -> w469
                      tunnel: w463 -> [_ w487 _ _ _ _ _]
                      tunnel: [w481 w485 w497 _ _ _ w512] -> w461
                      frame "fixsize" {
                        n247 = Not(x=w481) -> (.not. x?=w482:bool)
                        n248 = control-ref of="This VI"() -> (w483:refnum<vi>)
                        n249 = property class="VI"(reference=w483, "Front Panel.Resizeable"=w482) -> ()  [unwired: 1 in, 2 out]
                        "fixsize" <- w481
                      }
                      frame Default {
                        n250 = case shown="True" w487 {
                          tunnel: w486 -> [_ w495]
                          tunnel: [_ w491] -> w485
                          tunnel: w484 -> [_ w491]
                          frame False {
                          }
                          frame True {
                            n251 = control-ref of="This VI"() -> (w494:refnum<vi>)
                            n252 = control-ref of="reset"() -> (w493:refnum<vi>)
                            n253 = call "getPortAndIP.vi"("This Vi"=w494, "Device Name"=w495) -> ("port or service name"=w489:u16, "Remote Host"=w488:string)  [unwired: 1 in, 1 out]
                            n254 = local write "port or service name"(w489) -> ()
                            n255 = local write "Remote Host"(w488) -> ()
                            n256 = property class="Bool (strict)"(reference=w493, "Val(Sgnl)"=TRUE ("Value (Signaling)")) -> ()  [unwired: 1 in, 2 out]
                            n257 = call "ConnectionFGV.vi"("command"=enum16{"get", "set", "init"}."set", "Remote Host in"=w488, "port or service name in"=w489) -> ()  [unwired: 7 in, 2 out]
                          }
                        }
                      }
                      frame "ratio" {
                        n258 = property on="Image (IMAQ)" class="ImageControl"() -> ("ZoomSingle"=w496:cluster{"X":sgl, "Y":sgl})  [unwired: 2 in, 2 out]
                        n259 = local write "Zoom old"(w496) -> ()
                        "ratio(h)" <- w497
                      }
                      frame "Local Saving Path" {
                        n260 = control-ref of="localsavingpath"() -> (w499:refnum<vi>)
                        n261 = property class="Path"(reference=w499) -> (reference out=w502:refnum<vi>, "Value"=w503:path)  [unwired: 1 in, 1 out]
                        n262 = call "changePath.vi"("Local Saving in (h)"=w503) -> ("change (h)"=w501:bool, "Local Saving out (h)"=w500:path)  [unwired: 9 in]
                        n263 = case shown="True" w501 {
                          tunnel: w502 -> [_ w505]
                          tunnel: w500 -> [_ w504]
                          frame False {
                          }
                          frame True {
                            n264 = property class="Path"(reference=w505, "Val(Sgnl)"=w504) -> ()  [unwired: 1 in, 2 out]
                          }
                        }
                      }
                      frame "Binary", "Gradient", "Grayscale", "Rainbow", "Temperature" {
                        n265 = Scan From String(input string=w507, default 1=T6."Grayscale" ("Palette:Palette Type")) -> (output 1=w506:T6)  [unwired: 3 in, 3 out]
                        n266 = property on="Image (IMAQ)" class="ImageControl"("Palette Type"=w506) -> ()  [unwired: 2 in, 2 out]
                      }
                      frame "reset" {
                        n267 = control-ref of="reset"() -> (w510:refnum<vi>)
                        n268 = property class="Bool (strict)"(reference=w510, "Val(Sgnl)"=TRUE ("Value (Signaling)")) -> ()  [unwired: 1 in, 2 out]
                      }
                      frame "clear" {
                        n269 = control-ref of="reset"() -> (w514:refnum<vi>)
                        n270 = call "ClearBufferFGV.vi"("Command"=enum16{"set", "get", "init"}."set", "clear buffer"=w512) -> ()  [unwired: 9 in, 1 out]
                        n271 = property class="Bool (strict)"(reference=w514, "Val(Sgnl)"=TRUE ("Value (Signaling)")) -> ()  [unwired: 1 in, 2 out]
                      }
                    }
                    n272 = Set Menu Item Info(6:w461, 7:w468, 10:w471, 11:w462) -> ()  [unwired: 3 in, 2 out]
                  }
                }
              }
            }
          }
          event "time to wait (TCP)": Value Change {
            n273 = event-data() -> ("NewVal"=w524:i32)  [unwired: 1 in, 4 out]
            n274 = call "WaitFGV.vi"("Command"=enum16{"get", "set", "init"}."set", "milliseconds to wait"=w524) -> ()  [unwired: 9 in, 1 out]
          }
          event "Image (IMAQ)": Mouse Up {
            n275 = event-data() -> ()  [unwired: 1 in, 5 out]
            n276 = disable-structure shown="Disabled" {
              disable-tunnel: w528 -> [w543 _]
              disable-tunnel: w527 -> [w541 _]
              disable-tunnel: [w540 _] -> w526
              disable-tunnel: [w534 _] -> w525
              frame Disabled {
                n277 = local read "Zoom old"() -> (w531:cluster{"X":sgl, "Y":sgl})
                n278 = property on="Image (IMAQ)" class="ImageControl"() -> ("ZoomSingle"=w530:cluster{"X":sgl, "Y":sgl})  [unwired: 2 in, 2 out]
                n279 = property on="Image (IMAQ)" class="ImageControl"() -> ("ROI"=w542:T11)  [unwired: 2 in, 2 out]
                n280 = Unbundle By Name(w542) -> ("Global Rectangle"=w540:i32[])
                n281 = Unbundle By Name(w530) -> ("X"=w532:sgl)
                n282 = Unbundle By Name(w531) -> ("X"=w533:sgl)
                n283 = Not Equal?(x=w541, y=w540) -> (x != y?=w544:bool[])
                n284 = Empty Array?(array=w540) -> (empty?=w539:bool)
                n285 = Not Equal?(x=w532, y=w533) -> (x != y?=w529:bool)
                "Zoom changed" <- w529
                n286 = Empty Array?(array=w541) -> (empty?=w537:bool)
                n287 = Or Array Elements(Boolean array=w544) -> (logical OR=w535:bool)
                n288 = Not(x=w539) -> (.not. x?=w538:bool)
                n289 = case shown="True" w529 {
                  tunnel: w530 -> [_ w547]
                  frame False {
                  }
                  frame True {
                    n290 = local write "Zoom old"(w547) -> ()
                  }
                }
                n291 = case shown="True" w529 {
                  selector: w529 -> [_ w545]
                  frame False {
                  }
                  frame True {
                    n292 = control-ref of="resize"() -> (w546:refnum<vi>)
                    n293 = property class="Bool (strict)"(reference=w546, "Val(Sgnl)"=w545) -> ()  [unwired: 1 in, 2 out]
                  }
                }
                n294 = And(x=w537, y=w538) -> (x .and. y?=w536:bool)
                n295 = Or(x=w535, y=w536) -> (x .or. y?=w534:bool)
                n296 = case shown="True" w534 {
                  tunnel: w543 -> [_ _]
                  tunnel: w542 -> [_ w549]
                  frame False {
                  }
                  frame True {
                    n297 = call "ROI thickener.vi"("ROI Descriptor in"=w549) -> ("ROI Descriptor out"=w548:T14)  [unwired: 1 in, 1 out]
                    n298 = property on="Image (IMAQ)" class="ImageControl"("ROI"=w548) -> ()  [unwired: 2 in, 2 out]
                  }
                }
              }
              frame Enabled {
              }
            }
          }
        }
        "error out" <- w226
        n299 = call "IMAQ Copy"("Image Dst"=w200, "Image Src"=w201) -> ("Image Dst Out"=w199:T5)  [unwired: 4 in, 1 out]
        n300 = case shown="True" TRUE ("localanalysis") {
          tunnel: w201 -> [w249 w253]
          tunnel: [_ w259] -> w203
          tunnel: [w249 w254] -> w202
          tunnel: w199 -> [_ w252]
          frame False {
          }
          frame True {
            n301 = call "IMAQ Histograph"("Image"=w253) -> ("error out"=w263:errorcluster, "Mean Value"=→"Mean Value" →"Mean Value 2":sgl, "Histogram Graph"=→"histogram":T3)  [unwired: 7 in, 1 out]
            n302 = property on="Image (IMAQ)" class="ImageControl"() -> ("ROI"=w271:T11)  [unwired: 2 in, 2 out]
            n303 = call "IMAQ Convert ROI to Line"("ROI Descriptor"=w271) -> ("Line"=w270:T15)  [unwired: 8 in, 1 out]
            n304 = case shown="True" "lowpass" {
              tunnel: w253 -> [_ w278]
              tunnel: [w275 w280] -> w251
              tunnel: w252 -> [w275 w277]
              frame False {
              }
              frame True {
                n305 = call "IMAQ LowPass"("Image Src"=w278, "Size & Tolerance"="Size & Tolerance", "Image Dst"=w277) -> ("Image Dst Out"=w280:T5, "error out"=w276:errorcluster)  [unwired: 4 in]
                n306 = call <vilib>:"Clear Errors.vi"("error in (no error)"=w276) -> ()  [unwired: 6 in, 1 out]
              }
            }
            n307 = call "IMAQ Centroid"("error in (no error)"=w263, "Image"=w253) -> ("error out"=w273:errorcluster, "Centroid"=→"Centroid":cluster{"X Centroid":sgl, "Y Centroid":sgl})  [unwired: 2 in]
            n308 = Unbundle(w270) -> ("Start X"=w269:i32, "Start Y"=w268:i32, "End X"=w267:i32, "End Y"=w266:i32)
            n309 = Build Array(w269, w268, w267, w266) -> (w265:i32[])
            n310 = call "GetMaxCounts.vi"("New Image"=w251) -> ("Maximal Value"=w250:sgl, "Color"=w257:u32)
            "Max Counts" <- w250
            n311 = call "IMAQ LineProfile"("error in (no error)"=w273, "Line Coordinates"=w265, "Image"=w253) -> ("error out"=w259:errorcluster, "Line Graph"=→"lineout":cluster{"x0":sgl, "dx":sgl, "Pixels Line":sgl[]})  [unwired: 2 in, 2 out]
            "analysis error" <- w259
            n312 = property on="Max Counts" class="Slide (strict)"("Fill Color"=w257) -> ()  [unwired: 2 in, 2 out]
            n313 = Divide(x=256.0, y=w250) -> (x/y=w260:dbl)
            n314 = case shown="True" "autoscale" {
              tunnel: w251 -> [w284 w285]
              tunnel: w260 -> [_ w288]
              tunnel: [w284 w286] -> w254
              frame False {
              }
              frame True {
                n315 = call "IMAQ Multiply"("Image Src A"=w285, "Constant"=w288, "Image Dst"=w285) -> ("Image Dst Out"=w286:T5, "error out"=w287:errorcluster)  [unwired: 4 in]
                n316 = call <vilib>:"Clear Errors.vi"("error in (no error)"=w287) -> ()  [unwired: 6 in, 1 out]
              }
            }
            n317 = case shown="True" "beep if sat." {
              tunnel: w250 -> [_ w283]
              frame False {
              }
              frame True {
                n318 = Greater Or Equal?(x=w283, y="sat level") -> (x >= y?=w281:bool)
                n319 = case shown="True" w281 {
                  frame False {
                  }
                  frame True {
                    n320 = call <vilib>:"Beep.vi"() -> ()  [unwired: 12 in]
                  }
                }
              }
            }
          }
        }
        "Image (IMAQ)" <- w202
        n321 = control-ref of="error (h)"() -> (w235:refnum<vi>)
        n322 = control-ref of="error message"() -> (w242:refnum<vi>)
        n323 = Not(x="resize") -> (.not. x?=w230:bool)
        n324 = call "IMAQ GetImageSize"("Image"=w202, "error in (no error)"=w203) -> ("Y Resolution"=→"Y Resolution":i32, "X Resolution"=→"X Resolution":i32, "error out"=w204:errorcluster)  [unwired: 2 in]
        n325 = Preview Queue Element ("get stop queue value")(queue=w214, timeout in ms (-1)=5) -> (queue out=w212:refnum<queue>, element=w210:bool)  [unwired: 1 in, 2 out]
        n326 = Or(x=w211, y=w210) -> (x .or. y?=w209:bool)
        n327 = call <vilib>:"Clear Errors.vi"("error in (no error)"=w204) -> ()  [unwired: 6 in, 1 out]
        n328 = And(x=w230, y=w229) -> (x .and. y?=w228:bool)
        n329 = case shown="True" w209 {
          selector: w209 -> [_ w300]
          frame False {
          }
          frame True {
            n330 = call "StopFGV.vi"("Command"=enum16{"set", "get", "init"}."set", "Stop"=w300) -> ()  [unwired: 8 in, 2 out]
          }
        }
        n331 = Select(t=w239, s=w236, f=w237) -> (s? t:f=w238:i32[])
        n332 = call "clearErrorMessageGUI.vi"("millisecond timer value"=w243, "Boolean"=w241, "error message"=w242, "reference"=w235) -> ("millisecond timer value 2"=w244:u32)
        n333 = case shown="True" w228 {
          selector: w228 -> [w296 w298]
          tunnel: [w296 FALSE] -> w232
          frame False {
          }
          frame True {
            n334 = control-ref of="resize"() -> (w299:refnum<vi>)
            n335 = property class="Bool (strict)"(reference=w299, "Val(Sgnl)"=w298) -> ()  [unwired: 1 in, 2 out]
          }
        }
      }
      n336 = Call Chain() -> (call chain=w122:string[])
      n337 = Array Size(array=w122) -> (size(s)=w138:i32)
      n338 = Decrement(x=w138) -> (x-1=w137:i32)
      n339 = call "preset SQL Queries.vi"("Preset Query"=Preset_Query_Enum."GetItemLocatorIP") -> ("error out"=w132:errorcluster, "data"=w126:string[][])  [unwired: 8 in, 1 out]
      n340 = Random Number (0-1)() -> (number: 0 to 1=w117:dbl)
      n341 = Index Array(array=w122, index=w137) -> (element=w136:string)
      n342 = Number To Fractional String(number=w117) -> (F-format string=w115:string)  [unwired: 3 in]
      n343 = Index Array(array=w126, index (row) #1=w129, index (col) #1=0 ("disabled index (col)"), index (row) #2=w129, index (col) #2=1 ("disabled index (col)")) -> (element #1=w124:string, element #2=w125:string)
      n344 = Decimal String To Number(string=w125) -> (number=w131:i32)  [unwired: 2 in, 1 out]
      n345 = Match Pattern(string=w136, regular expression=".vi") -> (before substring=w134:string)  [unwired: 1 in, 3 out]
      n346 = To Unsigned Word Integer(number=w131) -> (unsigned 16bit integer=w130:u16)
      n347 = Concatenate Strings(w134, w115) -> (w116:string)
      n348 = call "TCP Write Alive 2.vi"("MultiCast Port"=w130, "Stopqueue"=w123, "address"=w124, "Name"=w116, "error in (no error)"=w132) -> ("error out"=w121:errorcluster)  [unwired: 8 in, 2 out]
      n349 = call "IMAQ Dispose"("Image"=w197) -> ()  [unwired: 5 in, 1 out]
      n350 = call "EventsFGV.vi"("Command"=enum16{"get", "init"}."get") -> ("New Event"=w162:T12)  [unwired: 9 in, 1 out]
      n351 = Unregister For Events(event registration refnum=w166, error in=w164) -> (error out=w165:errorcluster)
      n352 = Destroy User Event(user event=w162, error in=w165) -> (error out=w119:errorcluster)
      n353 = call <vilib>:"Clear Errors.vi"("error in (no error)"=w119) -> ("error out"=w118:errorcluster)  [unwired: 6 in]
      n354 = Lossy Enqueue Element(queue=w123, element=w120, error in (no error)=w118) -> (error out=w146:errorcluster)  [unwired: 3 out]
      n355 = call <vilib>:"Clear Errors.vi"("error in (no error)"=w146) -> ("error out"=w145:errorcluster)  [unwired: 6 in]
      n356 = Merge Errors(w145, w121) -> (w141:errorcluster)
      n357 = Flush Queue(queue=w123, error in (no error)=w141) -> (queue out=w139:refnum<queue>, error out=w144:errorcluster)  [unwired: 1 out]
      n358 = local read "connections (hidden)"() -> (w191:variant[])
      n359 = Release Queue(queue=w139, force destroy? (F)=TRUE, error in (no error)=w144) -> (error out=w142:errorcluster)  [unwired: 2 out]
      n360 = call <vilib>:"Clear Errors.vi"("error in (no error)"=w142) -> ("error out"=w140:errorcluster)  [unwired: 6 in]
      n361 = call "Close UDP AND TCP connections.vi"("error in"=w140, "appended array"=w191) -> ()  [unwired: 6 in]
    }
    frame #4 {
      n362 = flat-sequence {
        frame #0 {
          n363 = Wait (ms)(milliseconds to wait=u32 0) -> ()  [unwired: 1 out]
        }
        frame #1 {
          n364 = local write "stop"(FALSE ("stop")) -> ()
        }
        frame #2 {
          n365 = disable-structure shown="Disabled" {
            frame Disabled {
              n366 = control-ref of="This VI"() -> (w558:refnum<vi>)
              n367 = case shown="False" FALSE {
                tunnel: w558 -> [w559 w562]
                tunnel: [w559 w560] -> w557
                frame False {
                }
                frame True {
                  n368 = property class="VI" props=["Front Panel.Open"](reference=w562) -> (reference out=w561:refnum<vi>)  [unwired: 1 in, 2 out]
                  n369 = invoke class="VI" method="FP.Close"(reference=w561) -> (reference out=w560:refnum<vi>)  [unwired: 2 in, 2 out]
                }
              }
              n370 = Close Reference(reference=w557) -> ()  [unwired: 1 in, 1 out]
            }
            frame Enabled {
            }
          }
        }
      }
      n371 = control-ref of="Main  Control"() -> (w552:refnum<vi>)
      n372 = property class="TabCtl (strict)"(reference=w552, "Tab Location"=enum32{"Top", "Bottom", "Left", "Right"}."Bottom") -> ()  [unwired: 1 in, 2 out]
      n373 = property class="TabCtl (strict)"(reference=w552, "Tabs Visible?"=TRUE) -> ()  [unwired: 1 in, 2 out]
    }
  }
  n374 = property on="Image (array)" class="IntGraph (strict)"("Color Table"=u32[] [16777215, 8126719, 7864574, 7536895, 7274750, 6947071, 6684926, 6357247, 6095102, 5767423, 5505278, 5177599, 4915454, 4587775, 4325630, 3997951, 3735806, 3408127, 3145982, 2818303, 2556158, 2228479, 1966334, 1638655, 1376510, 1048831, 786686, 459007, 196862, 767, 1790, 3071, 4094, 5375, 6398, 7679, 8702, 9983, 11006, 12287, 13310, 14591, 15614, 16895, 17918, 19199, 20222, 21503, 22526, 23807, 24830, 26111, 27134, 28415, 29438, 30719, 31486, 33023, 33790, 35327, 36094, 37631, 38398, 39935, 40702, 42239, 43006, 44543, 45310, 46847, 47614, 49151, 49918, 51455, 52222, 53759, 54526, 56063, 56830, 58367, 59134, 60671, 61694, 62975, 63998, 65279, 65274, 65527, 65265, 65518, 65256, 65509, 65247, 65500, 65238, 65491, 65229, 65482, 65220, 65473, 65211, 65464, 65202, 65455, 65193, 65446, 65184, 65437, 65175, 65428, 65166, 65419, 65157, 65410, 65149, 65401, 65140, 65392, 65131, 65383, 65122, 65374, 65113, 65365, 65104, 65356, 65095, 65347, 65086, 65338, 65077, 65329, 65068, 65320, 65059, 65311, 65050, 65302, 65041, 65293, 65032, 65284, 130560, 392960, 720384, 982784, 1310208, 1572608, 1900032, 2162432, 2489856, 2752256, 3079680, 3342080, 3669504, 3931904, 4259328, 4521728, 4849152, 5111552, 5438976, 5701376, 6028800, 6291200, 6618624, 6881024, 7208448, 7470848, 7798272, 8126208, 8322560, 8716032, 8912384, 9305856, 9502208, 9895680, 10092032, 10485504, 10681856, 11075328, 11271680, 11665152, 11861504, 12254976, 12451328, 12844800, 13041152, 13434624, 13630976, 14024448, 14220800, 14614272, 14810624, 15204096, 15400448, 15793920, 15990272, 16383744, 16580096, 16776192, 16709376, 16773888, 16707072, 16771584, 16704768, 16769280, 16702464, 16766976, 16700160, 16764672, 16697856, 16762368, 16695552, 16760064, 16693248, 16757760, 16690944, 16755456, 16688640, 16753152, 16686336, 16750848, 16684032, 16748544, 16681728, 16746240, 16679680, 16743936, 16677376, 16741632, 16675072, 16739328, 16672768, 16737024, 16670464, 16734720, 16668160, 16732416, 16665856, 16730112, 16663552, 16727808, 16661248, 16725504, 16658944, 16723200, 16656640, 16720896, 16654336, 16718592, 16652032, 16716288, 16649728, 16713984, 16712960, 0] ("256 rainbow")) -> ()  [unwired: 2 in, 2 out]
  n375 = control-ref of="This VI"() -> (w3:refnum<vi>)
  n376 = disable-structure "Factory Pattern: Enable plugin" shown="RUN_TIME_ENGINE==True" {
    disable-tunnel: w2 -> [_ w567]
    disable-tunnel: w3 -> [w563 w566]
    disable-tunnel: [_ w565] -> _
    disable-tunnel: [w563 w564] -> w1
    frame condition #0 (active) {
    }
    frame condition #1 {
      n377 = property class="VI"(reference=w566, error in=w567, "Front Panel.Open"=FALSE) -> (reference out=w564:refnum<vi>, error out=w565:errorcluster)
    }
  }
  n378 = Close Reference(reference=w1) -> ()  [unwired: 1 in, 1 out]
